vi "Demodlator.vi"(8 "error in (no error)":errorcluster, 10 "Waveform in":waveform(dbl), 11 "ISO 14443 A DOWN in":refnum<class "ISO 14443 A DOWN.lvclass">) -> (0 "error out":errorcluster, 2 "Waveform out":waveform(dbl), 3 "ISO 14443 A DOWN out":refnum<class "ISO 14443 A DOWN.lvclass">)   [LabVIEW 2019, in "ISO 14443 A DOWN.lvclass"]
uses:
  ISO 14443 A DOWN.lvclass
  TypeDef/Store.ctl
  ISO 14443 A DOWN.lvclass/ISO 14443 A DOWN.ctl
  <vilib>/addons/Modulation/Analog/support/mod_Set Error Source.vi
  <vilib>/addons/Modulation/Digital/Support/Common/Validators/mod_Generate Filter Coefficients Validate.vi
  <vilib>/addons/Modulation/Digital/General/subVIs/mod_Generate Filter Coefficients.vi
  <vilib>/addons/Modulation/Digital/General/MT Generate ASK system parameters (M).vi
  <vilib>/addons/Modulation/Analog/MT Demodulate AM (DSB).vi
  <vilib>/addons/Modulation/Analog/MT Downconvert Passband (Real).vi
  <vilib>/addons/Modulation/niAMT.lvlib
  <vilib>/addons/Modulation/niDMT.lvlib
  RFID system.lvclass
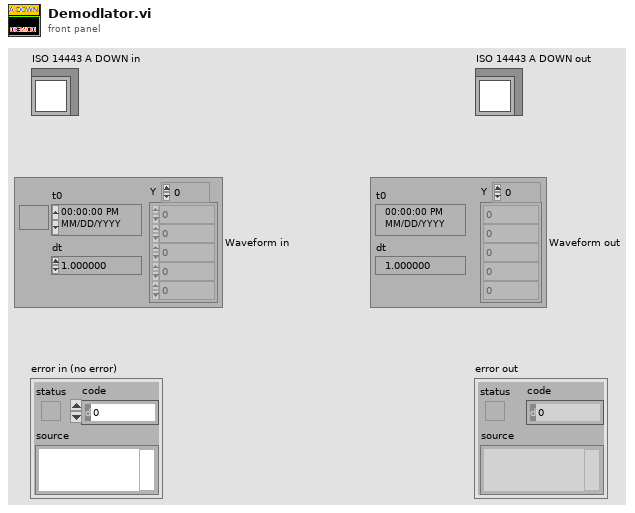
[diagram p1: front panel]
types:
  T1 = typedef "Store.ctl" = enum16{"envelope", "noise", "demSubCar", "CH_frame", "Decode", "demodulate", "in", "out", "sum", "subCarrier", "frame", "command", "encode", "modulate", "encode_UP", "modulate_up", "demod_up", "envelop_up", "sum_up", "out_up", "in_up"}
  T2 = enum16{"none", "Raised Cosine", "Root Raised Cos", "Gaussian"}
  T3 = enum16{"FSK", "PSK", "QAM", "MSK", "PAM", "ASK", "CPM"}
  T4 = cluster{"passband ripple (dB)":dbl, "stopband start (Hz)":dbl, "stopband gain (dB)":dbl, "compute filter stopband ? (T)":bool}
  T5 = typedef "niAMT.lvlib/Complex Data Waveform.ctl" = cluster{"t0":dbl, "dt":dbl, "Y":cdb[]}
  T6 = cluster{"samples per symbol (16)":i32, "symbol map":cdb[]}
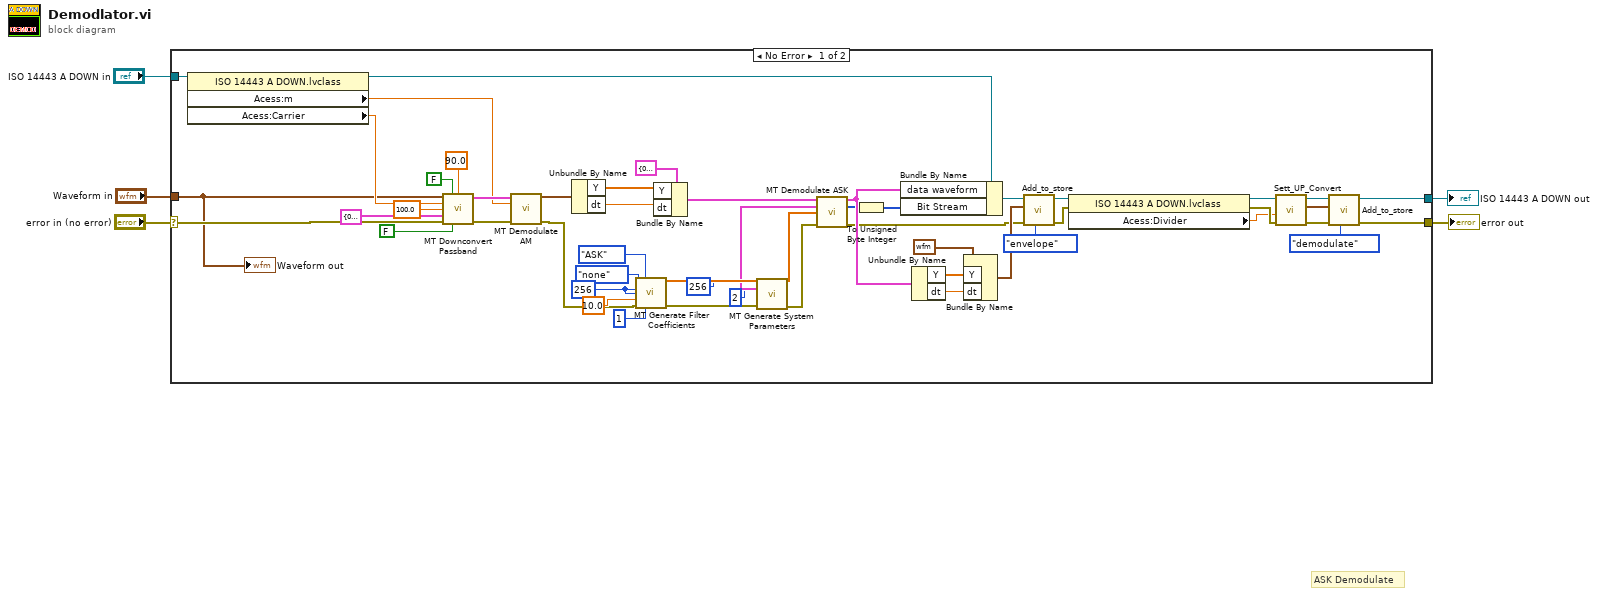
[diagram p0: block diagram]
diagram:
  # "ASK Demodulate"
  n1 = case shown="No Error" "error in (no error)" {
    selector: "error in (no error)" -> [w33 w58]
    tunnel: [w18 w58] -> w4
    tunnel: "ISO 14443 A DOWN in" -> [w56 w57]
    tunnel: [w19 w57] -> w2
    tunnel: "Waveform in" -> [w6 _]
    frame No Error {
      w39 = 256 ("pulse shaping samples per symbol (16)")
      n2 = property class="ISO 14443 A DOWN.lvclass"(reference=w56) -> (reference out=w30:refnum<class "ISO 14443 A DOWN.lvclass">, "Acess:m"=w10:dbl, "Acess:Carrier"=w9:dbl)  [unwired: 1 in, 1 out]
      n3 = call-poly <vilib>:"MT Downconvert Passband.vi"("Waveform"=w6, "reset? (F)"=FALSE, "initial phase (deg)"=90.0, "carrier frequency (Hz)"=w9, "passband bandwidth (Hz)"=100.0, "advanced filter parameters"=T4 {"passband ripple (dB)"=0.01, "stopband start (Hz)"=0.0, "stopband gain (dB)"=-96.0, "compute filter stopband ? (T)"=TRUE}, "error in (no error)"=w33, "enable filter (T)"=FALSE) -> ("downconverted waveform (complex baseband)"=w55:T5, "error out"=w54:errorcluster)  [unwired: 4 in, 2 out]
      n4 = call-poly <vilib>:"MT Demodulate AM.vi"("AM modulated waveform"=w55, "modulation index"=w10, "error in (no error)"=w54) -> ("AM demodulated waveform"=w34:waveform(dbl), "error out"=w32:errorcluster)  [unwired: 10 in, 1 out]
      n5 = Unbundle By Name(w34) -> ("Y"=w46:dbl[], "dt"=w47:dbl)
      n6 = call <vilib>:"MT Generate Filter Coefficients.vi"("pulse shaping filter (none)"=T2."none", "modulation type"=T3."ASK", "pulse shaping samples per symbol (16)"=w39, "matched samples per symbol (16)"=w39, "filter parameter"=10.0, "error in (no error)"=w32, "filter length (symbols)"=1) -> ("pulse shaping filter coefficients"=w45:dbl[], "error out"=w43:errorcluster)  [unwired: 7 out]
      n7 = Bundle By Name(cluster=cluster{"t0":dbl, "dt":dbl, "Y":dbl[]} {"t0"=0.0, "dt"=0.0, "Y"=[]} ("AM modulated waveform"), "Y"=w46, "dt"=w47) -> (w48:cluster{"t0":dbl, "dt":dbl, "Y":dbl[]})
      n8 = call-poly <vilib>:"MT Generate System Parameters.vi"("samples per symbol (16)"=256, "M-ASK (2)"=2, "error in (no error)"=w43) -> ("ASK system parameters"=w44:T6, "error out"=w31:errorcluster)  [unwired: 11 out]
      n9 = call <vilib>:"MT Demodulate ASK.vi"("input complex waveform"=w48, "ASK system parameters"=w44, "matched filter coefficients"=w45, "error in (no error)"=w31) -> ("recovered complex waveform"=w25:T5, "output bit stream"=w8:i8[], "error out"=w23:errorcluster)  [unwired: 7 in, 2 out]
      n10 = To Unsigned Byte Integer(number=w8) -> (unsigned 8bit integer=w7:u8[])
      n11 = Bundle By Name(cluster=w30, "data waveform"=w25, "Bit Stream"=w7) -> (w29:refnum<class "ISO 14443 A DOWN.lvclass">)
      n12 = Unbundle By Name(w25) -> ("Y"=w27:cdb[], "dt"=w26:dbl)
      n13 = Bundle By Name(cluster=waveform(cdb) {"t0"=timestamp(0 s since 1904-01-01), "dt"=1.0, "Y"=[]} ("waveform"), "Y"=w27, "dt"=w26) -> (w24:waveform(cdb))
      n14 = call "Add_to_store.vi"("Store"=Store."envelope", "error in (no error)"=w23, "Waveform"=w24, "RFID system in"=w29) -> ("error out"=w13:errorcluster, "RFID system out"=w21:refnum<class "ISO 14443 A DOWN.lvclass">)  [unwired: 6 in]
      n15 = property class="ISO 14443 A DOWN.lvclass"(reference=w21, error in=w13) -> (reference out=w14:refnum<class "ISO 14443 A DOWN.lvclass">, error out=w12:errorcluster, "Acess:Divider"=w11:dbl)
      n16 = call-dynamic "Sett_UP_Convert.vi"("error in (no error)"=w12, "Divider(1)"=w11, "ISO 14443 A DOWN in"=w14) -> ("error out"=w17:errorcluster, "Waveform"=w16:waveform(dbl), "ISO 14443 A DOWN out"=w20:refnum<class "ISO 14443 A DOWN.lvclass">)  [unwired: 6 in]
      n17 = call "Add_to_store.vi"("Store"=Store."demodulate", "error in (no error)"=w17, "Waveform"=w16, "RFID system in"=w20) -> ("error out"=w18:errorcluster, "RFID system out"=w19:refnum<class "ISO 14443 A DOWN.lvclass">)  [unwired: 6 in]
      "Waveform out" <- w6
    }
    frame Error {
    }
  }
  "error out" <- w4
  "ISO 14443 A DOWN out" <- w2
